vi "Check Status.vi"(8 "error in (no error)":errorcluster, 11 "Panel Control Counter in":refnum<class "Panel Control Counter.lvclass">) -> (0 "error out":errorcluster, 2 "Fully Released?":bool)   [LabVIEW 2020, in "Panel.lvlib" / "Panel Control Counter.lvclass"]
doc: "Checks if the Panel Control Counter is fully released.\n\n----\nPlease see the following web address for additional documentation and tutorial information:\nhttp://www.mooregoodideas.com/mgi-panel-manager/\n\nAuthor: Derek Trepanier\n\nCopyright (c) 2018, Moore Good Ideas, Inc.\n\nAll rights reserved.\n\nRedistribution and use in source and binary forms, with or without modification, are permitted provided that the following conditions are met:\n\n * Redistributions of source code must retain the above copyright notice, this list of conditions and the following disclaimer.\n * Redistributions in binary form must reproduce the above copyright notice, this list of conditions and the following disclaimer in the documentation and/or other materials provided with the distribution.\n * Neither the name of Moore Good Ideas, Inc. nor the names of its contributors may be used to endorse or promote products derived from this software without specific prior written permission.\n\nTHIS SOFTWARE IS PROVIDED BY THE COPYRIGHT HOLDERS AND CONTRIBUTORS \"AS IS\" AND ANY EXPRESS OR IMPLIED WARRANTIES, INCLUDING, BUT NOT LIMITED TO, THE IMPLIED WARRANTIES OF MERCHANTABILITY AND FITNESS FOR A PARTICULAR PURPOSE ARE DISCLAIMED. IN NO EVENT SHALL THE COPYRIGHT OWNER OR CONTRIBUTORS BE LIABLE FOR ANY DIRECT, INDIRECT, INCIDENTAL, SPECIAL, EXEMPLARY, OR CONSEQUENTIAL DAMAGES (INCLUDING, BUT NOT LIMITED TO, PROCUREMENT OF SUBSTITUTE GOODS OR SERVICES; LOSS OF USE, DATA, OR PROFITS; OR BUSINESS INTERRUPTION) HOWEVER CAUSED AND ON ANY THEORY OF LIABILITY, WHETHER IN CONTRACT, STRICT LIABILITY, OR TORT (INCLUDING NEGLIGENCE OR OTHERWISE) ARISING IN ANY WAY OUT OF THE USE OF THIS SOFTWARE, EVEN IF ADVISED OF THE POSSIBILITY OF SUCH DAMAGE."
uses:
  <vilib>/MGI/Panel Manager/Panel/Panel Control Counter/Panel Control Counter.lvclass
  <vilib>/MGI/Panel Manager/Panel/Panel Control Counter/Panel Control Counter.lvclass/Panel Control Counter.ctl
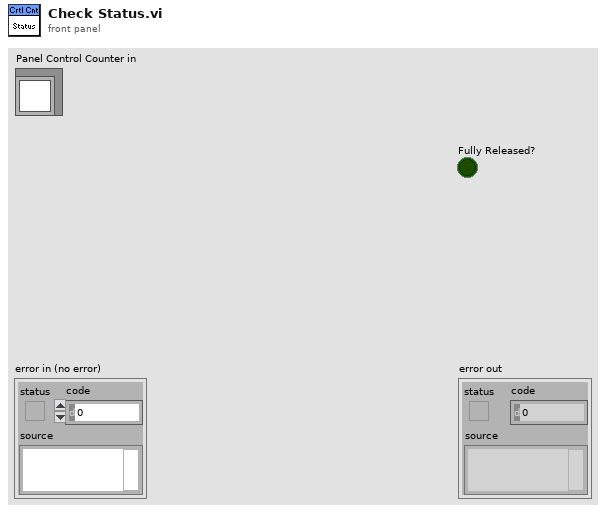
[diagram p1: front panel]
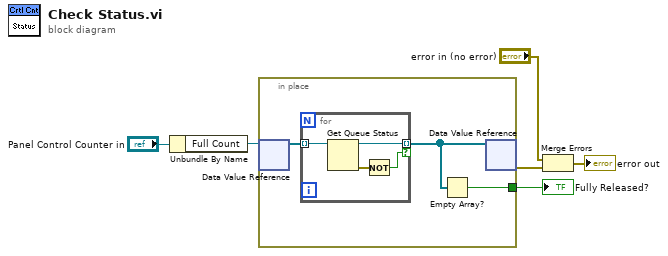
[diagram p0: block diagram]
diagram:
  n1 = Unbundle By Name("Panel Control Counter in") -> ("Full Count"=w4:refnum<data-value>)
  n2 = in-place {
    in-place-border: [w7] -> w3
    n3 = in-place-dvr #1(w4) -> (w9:refnum<queue>[])  [unwired: 1 out]
    n4 = for {
      tunnel: [w12] -> w8 mode=indexing if=w10
      tunnel: w9 -> [w13] mode=indexing
      n5 = Get Queue Status(queue=w13) -> (queue out=w12:refnum<queue>, error out=w11:errorcluster)  [unwired: 2 in, 6 out]
      n6 = Not(x=w11) -> (.not. x?=w10:bool)
    }
    n7 = Empty Array?(array=w8) -> (empty?=w7:bool)
    n8 = in-place-dvr #1(w8) -> (w1:errorcluster)  [unwired: 1 out]
  }
  "Fully Released?" <- w3
  n9 = Merge Errors("error in (no error)", w1) -> (→"error out":errorcluster)
